vi "AOTFInit.vi"(1 "error in (no error)":errorcluster) -> (0 "error out":errorcluster)   [LabVIEW 2009]
uses:
  AOTFSettings.ctt
  <vilib>/Utility/config.llb/NI_LVConfig.lvlib
panel:
  out "AOTF Setting":T1={"Laser 1 Output Channel"="5", "AOTF  1 Output Voltage"=2.0, "Laser 2 Output Channel"="6", "AOTF  2 Output Voltage"=5.0, "Laser 3 Output Channel"="1", "AOTF  3 Output Voltage"=0.0, "Pixel per Cycle"=0, "Time per Cycle  / ms"=10.0, "Laser 4 Output Channel"="1", "AOTF  4 Output Voltage"=0.0, "Laser 5 Output Channel"="1", "AOTF 5 Output Voltage "=0.0, "Laser 6 Output Channel"="1", "AOTF  6 Output Voltage "=0.0, "Laser 7 Output Channel"="1", "AOTF 7 Output Voltage "=0.0, "Laser 8 Output Channel"="1", "AOTF  8 Output Voltage "=0.0, "AOTF  1 Frequency"=84.0, "AOTF  2 Frequency"=88.0, "AOTF  3  Frequency"=94.0, "AOTF  4 Frequency"=101.0, "AOTF 5 Frequency"=109.0, "AOTF  6 Frequency"=119.0, "AOTF 7  Frequency"=127.0, "AOTF  8 Frequency"=137.0, "AOTF  1 Amplitude"=84.0, "AOTF  2 Amplitude"=88.0, "AOTF  3  Amplitude"=94.0, "AOTF  4 Amplitude"=101.0, "AOTF 5 Amplitude"=109.0, "AOTF  6 Amplitude"=119.0, "AOTF 7 Amplitude  "=127.0, "AOTF  8 Amplitude"=137.0} {"AOTF  8 Amplitude" format="%.2f"; "AOTF 7 Amplitude" format="%.2f"; "AOTF  6 Amplitude" format="%.2f"; "AOTF 5 Amplitude" format="%.2f"; "AOTF  4 Amplitude" format="%.2f"; "AOTF  3  Amplitude" min=0.0 max=10000000.0 format="%.2f"; "AOTF  2 Amplitude" min=0.0 max=10000000.0 format="%.2f"; "AOTF  1 Amplitude" min=0.0 max=1000000.0 format="%.2f"; "AOTF  8 Frequency" format="%.2f"; "AOTF 7  Frequency" format="%.2f"; "AOTF  6 Frequency" format="%.2f"; "AOTF 5 Frequency" format="%.2f"; "AOTF  4 Frequency" format="%.2f"; "AOTF  3  Frequency" min=0.0 max=10000000.0 format="%.2f"; "AOTF  2 Frequency" min=0.0 max=10000000.0 format="%.2f"; "AOTF  1 Frequency" min=0.0 max=1000000.0 format="%.2f"; "AOTF  8 Output Voltage" format="%.2f"; "AOTF 7 Output Voltage" format="%.2f"; "AOTF  6 Output Voltage" format="%.2f"; "AOTF 5 Output Voltage" format="%.2f"; "AOTF  4 Output Voltage" format="%.2f"; "Time per Cycle  / ms" format="%#.3f"; "AOTF  3 Output Voltage" min=0.0 max=10.0 format="%.2f"; "AOTF  2 Output Voltage" min=0.0 max=10.0 format="%.2f"; "AOTF  1 Output Voltage" min=0.0 max=10.0 format="%.2f"}
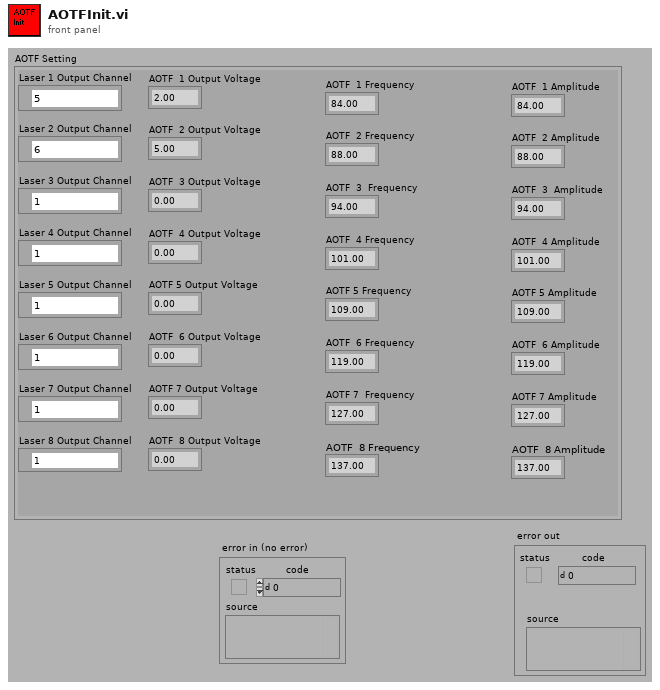
[diagram p1: front panel]
types:
  T1 = typedef "AOTFSettings.ctt" = cluster{"Laser 1 Output Channel":tag, "AOTF  1 Output Voltage":dbl, "Laser 2 Output Channel":tag, "AOTF  2 Output Voltage":dbl, "Laser 3 Output Channel":tag, "AOTF  3 Output Voltage":dbl, "Pixel per Cycle":u16, "Time per Cycle  / ms":dbl, "Laser 4 Output Channel":tag, "AOTF  4 Output Voltage":dbl, "Laser 5 Output Channel":tag, "AOTF 5 Output Voltage ":dbl, "Laser 6 Output Channel":tag, "AOTF  6 Output Voltage ":dbl, "Laser 7 Output Channel":tag, "AOTF 7 Output Voltage ":dbl, "Laser 8 Output Channel":tag, "AOTF  8 Output Voltage ":dbl, "AOTF  1 Frequency":dbl, "AOTF  2 Frequency":dbl, "AOTF  3  Frequency":dbl, "AOTF  4 Frequency":dbl, "AOTF 5 Frequency":dbl, "AOTF  6 Frequency":dbl, "AOTF 7  Frequency":dbl, "AOTF  8 Frequency":dbl, "AOTF  1 Amplitude":dbl, "AOTF  2 Amplitude":dbl, "AOTF  3  Amplitude":dbl, "AOTF  4 Amplitude":dbl, "AOTF 5 Amplitude":dbl, "AOTF  6 Amplitude":dbl, "AOTF 7 Amplitude  ":dbl, "AOTF  8 Amplitude":dbl}
  T2 = typedef "NI_LVConfig.lvlib/Config Data RefNum.ctl" = refnum<k1>
  T3 = cluster{"Laser 1 Output Channel":tag, "AOTF  1 Output Voltage":dbl, "Laser 2 Output Channel":tag, "AOTF  2 Output Voltage":dbl, "Laser 3 Output Channel":tag, "AOTF  3 Output Voltage":dbl, "Pixel per Cycle":u16, "Time per Cycle  / ms":dbl, "Laser 4 Output Channel":tag, "AOTF  4 Output Voltage":dbl, "Laser 5 Output Channel":tag, "AOTF 5 Output Voltage ":dbl, "Laser 6 Output Channel":tag, "AOTF  6 Output Voltage ":dbl, "Laser 7 Output Channel":tag, "AOTF 7 Output Voltage ":dbl, "Laser 8 Output Channel":tag, "AOTF  8 Output Voltage ":dbl, "AOTF  1 Frequency":dbl, "AOTF  2 Frequency":dbl, "AOTF  3  Frequency":dbl, "AOTF  4 Frequency":dbl, "AOTF 5 Frequency":dbl, "AOTF  6 Frequency":dbl, "AOTF 7  Frequency":dbl, "AOTF  8 Frequency":dbl, "AOTF  1 Amplitude":dbl, "AOTF  2 Amplitude":dbl, "AOTF  3  Amplitude":dbl, "AOTF  4 Amplitude":dbl, "AOTF 5 Amplitude":dbl, "AOTF  6 Amplitude":dbl, "AOTF 7 Amplitude  ":dbl, "AOTF  8 Amplitude":dbl}
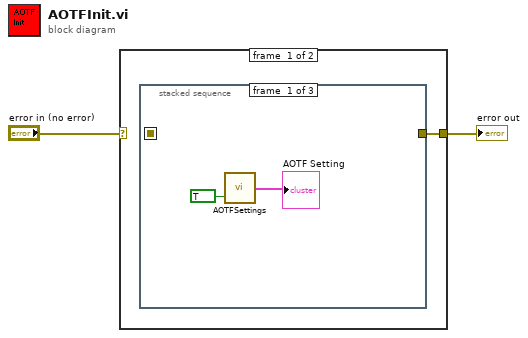
[diagram p0: block diagram]
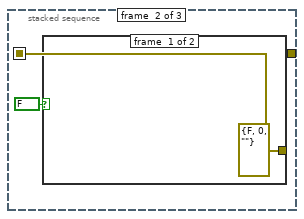
[diagram p2: hidden frame]
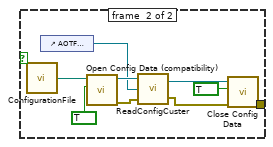
[diagram p3: hidden frame]
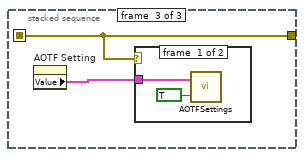
[diagram p4: hidden frame]
diagram:
  n1 = case shown="No Error" "error in (no error)" {
    selector: "error in (no error)" -> [_ w22]
    tunnel: [w3 w22] -> w1
    frame #0 {
      n2 = stacked-sequence {
        seq-local: [_ w7 _] -> [_ _ w18]
        tunnel: [_ _ w18] -> w3
        frame #0 {
          n3 = call "AOTFSettings.vi"("Get/Set"=TRUE) -> ("AOTF Setting (Output)"=→"AOTF Setting":T1)  [unwired: 1 in]
        }
        frame #1 {
          n4 = case shown="True" FALSE {
            tunnel: [errorcluster {"status"=FALSE, "code"=0, "source"=""} ("error out") w13] -> w7
            frame #0 {
            }
            frame #1 {
              n5 = call "ConfigurationFile.vi"() -> ("Configuration File (output)"=w12:path)  [unwired: 2 in]
              n6 = control-ref of="AOTF Setting"() -> (w9:refnum<vi>)
              n7 = call <vilib>:"Open Config Data (compatibility).vi"("create file if necessary (T)"=TRUE ("create file if necessary? (T)"), "configuration file path"=w12) -> ("error out"=w15:errorcluster, "refnum"=w16:T2)  [unwired: 7 in, 1 out]
              n8 = call "ReadConfigCuster.vi"("error in (no error)"=w15, "Ctrl Reference"=w9, "ConfigFile (input)"=w16) -> ("error out"=w10:errorcluster, "ConfigFile (output)"=w11:T2)
              n9 = call "Close Config Data.vi"("error in (no error)"=w10, "write configuration file? (T)"=TRUE ("write configuration file? (F)"), "refnum"=w11) -> ("error out"=w13:errorcluster)  [unwired: 8 in]
            }
          }
        }
        frame #2 {
          n10 = property on="AOTF Setting" class="Clust (strict)"() -> ("Value"=w19:T3)  [unwired: 2 in, 2 out]
          n11 = case shown="No Error" w18 {
            tunnel: w19 -> [w20 _]
            frame #0 {
              n12 = call "AOTFSettings.vi"("Get/Set"=TRUE ("Set"), "AOTF Setting (Input)"=w20) -> ()  [unwired: 1 out]
            }
            frame #1 {
            }
          }
        }
      }
    }
    frame #1 {
    }
  }
  "error out" <- w1
